vi "Stop Core.vi"(10 "final error code":i32, 11 "Dispatcher in":refnum<class "Dispatcher.lvclass">) -> (3 "Dispatcher out":refnum<class "Dispatcher.lvclass">)   [LabVIEW 2013, in "Dispatcher.lvclass"]
doc: "(<B>Filename</B>: Actor Framework.lvlib:Actor.lvclass:Stop Core.vi)\n\nDefines what the actor does before it stops. Use the <B>final error code</B> input to determine whether the actor shut down in response to an error.\n\nBy default, this method does nothing. A descendant class may override it to define behavior, such as shutting down any processes the actor initiated in its override of the Actor Core method."
uses:
  Dispatcher.lvclass
  <vilib>/ActorFramework/Actor/Actor.lvclass
  Dispatcher.lvclass/Dispatcher.ctl
  <vilib>/ActorFramework/Stop Msg/Stop Msg.lvclass/Stop Msg.ctl
  <vilib>/ActorFramework/Message Enqueuer/Message Enqueuer.lvclass/Message Enqueuer.ctl
  <vilib>/ActorFramework/Stop Msg/Send Emergency Stop.vi
  <vilib>/ActorFramework/Stop Msg/Send Normal Stop.vi
  <vilib>/ActorFramework/Message Enqueuer/Enqueue Critical.vi
  <vilib>/ActorFramework/Message Enqueuer/Enqueue.vi
  <vilib>/ActorFramework/Message Priority Queue/Priority Enqueue.vi
  <vilib>/ActorFramework/Stop Msg/Stop Msg.lvclass
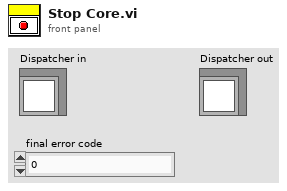
[diagram p1: front panel]
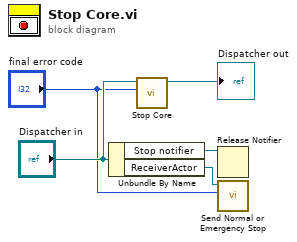
[diagram p0: block diagram]
diagram:
  n1 = Unbundle By Name("Dispatcher in") -> ("Stop notifier"=w3:refnum<notifier>, "ReceiverActor"=w2:refnum<class "Message Enqueuer.lvclass">)
  n2 = call-parent "Stop Core.vi"("final error code"="final error code", "Actor in"="Dispatcher in") -> ("Actor out"=→"Dispatcher out":refnum<class "Dispatcher.lvclass">)  [unwired: 9 in]
  n3 = Release Notifier(notifier=w3) -> ()  [unwired: 2 in, 3 out]
  n4 = call <vilib>:"Send Normal or Emergency Stop.vi"("final error code"="final error code", "Message Enqueuer"=w2) -> ()  [unwired: 9 in, 1 out]
